vi "4110_Volt _Chan Config Dialog.vi"(8 "error in (no error)":errorcluster, 11 "Data Entry Limits:Maximum":dbl) -> (0 "error out":errorcluster, 1 "sense (out)":T1=1008 items=["Local"=1008, "Remote"=1009], 2 "Current Limit (out)":dbl, 3 "Initial Voltage Value (out)":dbl, 4 "Cancel (out)":bool, 5 "Number of Voltage Output Channels to Add? (out)":i16)   [LabVIEW 2009, in "NI PXI-4110 Programmable Power Supply Custom Device.lvlib"]
uses:
  <instrlib>/niDCPower/nidcpower.llb/niDCPower Sense.ctl
  NI PXI-4110 Programmable Power Supply Custom Device.lvlib
panel:
  in  "Cancel":bool
  in  "OK Button":bool
  in  "Current Limit":dbl format="%.4f"
  in  "Initial Voltage Value":dbl
  in  "sense":T1=1008 caption="Sense" items=["Local"=1008, "Remote"=1009]
  in  "Number of Voltage Output Channels to Add?":i16
  # "Voltage Channels"
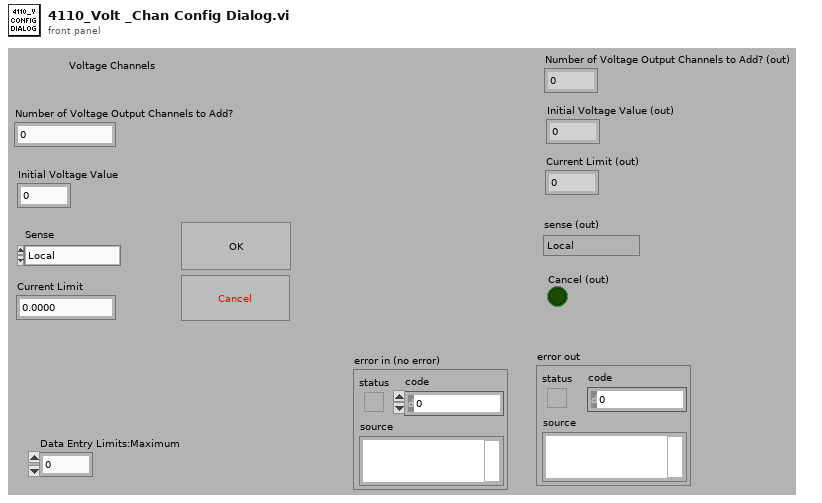
[diagram p1: front panel]
types:
  T1 = typedef "niDCPower Sense.ctl" = i32
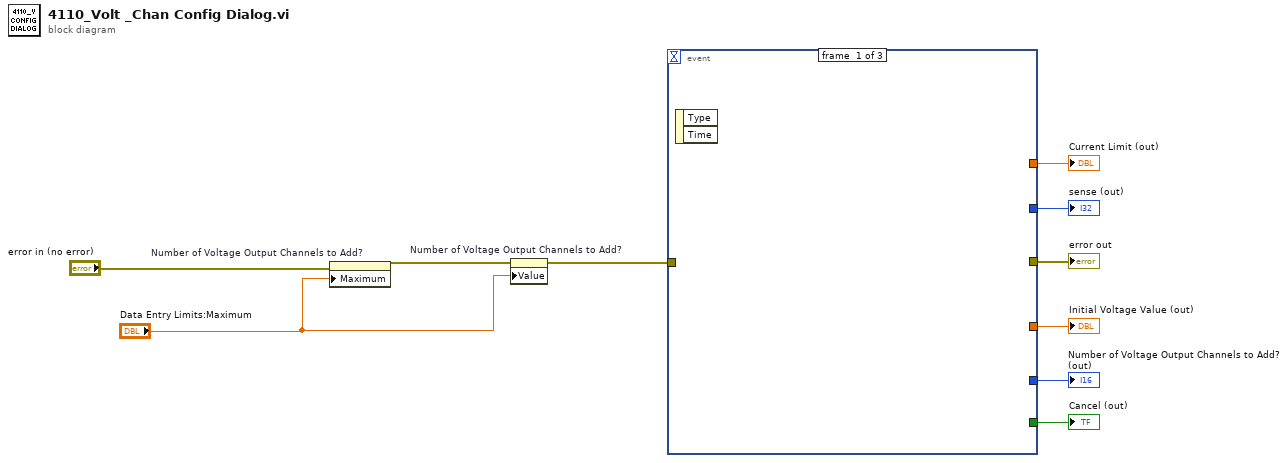
[diagram p0: block diagram]
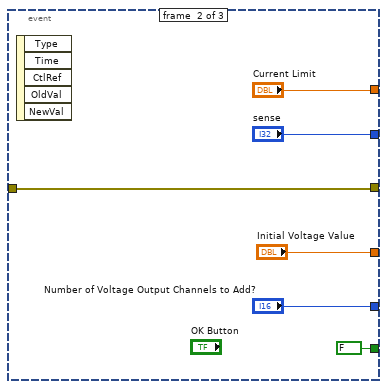
[diagram p2: hidden frame]
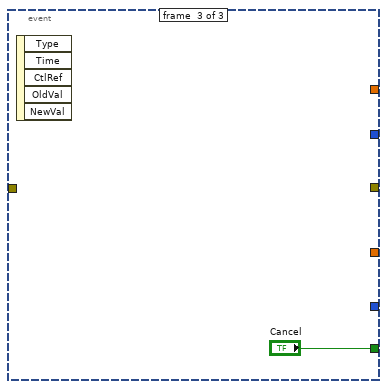
[diagram p3: hidden frame]
diagram:
  n1 = property on="Number of Voltage Output Channels to Add?" class="DigNum (strict)"(error in="error in (no error)", "Maximum"="Data Entry Limits:Maximum") -> (error out=w10:errorcluster)  [unwired: 1 in, 1 out]
  n2 = property on="Number of Voltage Output Channels to Add?" class="DigNum (strict)"(error in=w10, "Value"="Data Entry Limits:Maximum") -> (error out=w8:errorcluster)  [unwired: 1 in, 1 out]
  n3 = event shown="[1] \"OK Button\": Value Change" {
    selector: _ -> [_ _ _]
    dyn-events: _ -> [_ _ _]
    timeout: _ -> [_ _ _]
    tunnel: [_ "Current Limit" _] -> w6
    tunnel: [_ "sense" _] -> w5
    tunnel: [_ "Initial Voltage Value" _] -> w4
    tunnel: w8 -> [_ w13 _]
    tunnel: [_ w13 _] -> w7
    tunnel: [_ FALSE ("Cancel") "Cancel"] -> w3
    tunnel: [_ "Number of Voltage Output Channels to Add?" _] -> w1
    event #0 {
      n4 = event-data() -> ()  [unwired: 1 in, 2 out]
    }
    event #1 {
      n5 = event-data() -> ()  [unwired: 1 in, 5 out]
    }
    event #2 {
      n6 = event-data() -> ()  [unwired: 1 in, 5 out]
    }
  }
  "error out" <- w7
  "Current Limit (out)" <- w6
  "sense (out)" <- w5
  "Initial Voltage Value (out)" <- w4
  "Cancel (out)" <- w3
  "Number of Voltage Output Channels to Add? (out)" <- w1
